vi "DeadbandFilter.vi"(8 "guardband value":dbl=0.1 format="%#_13g", 10 "JoystickAxis":dbl) -> (2 "FilteredJoystickAxis":dbl)   [LabVIEW 2017]
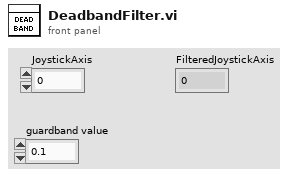
[diagram p1: front panel]
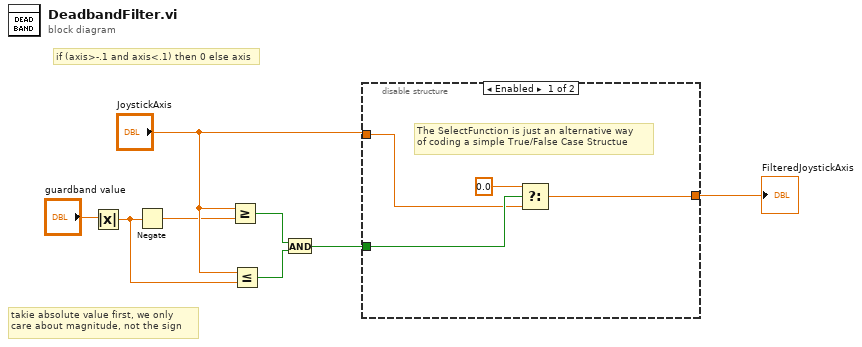
[diagram p0: block diagram]
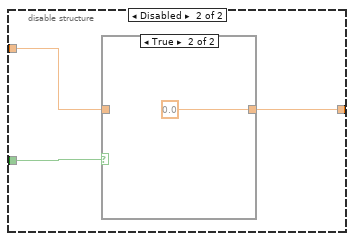
[diagram p2: hidden frame]
diagram:
  # "takie absolute value first, we only \ncare about magnitude, not the sign"
  # "if (axis>-.1 and axis<.1) then 0 else axis"
  n1 = Absolute Value(x="guardband value") -> (abs(x)=w1:dbl)
  n2 = Negate(x=w1) -> (-x=w2:dbl)
  n3 = Greater Or Equal?(x="JoystickAxis", y=w2) -> (x >= y?=w7:bool)
  n4 = Less Or Equal?(x="JoystickAxis", y=w1) -> (x <= y?=w8:bool)
  n5 = And(x=w7, y=w8) -> (x .and. y?=w6:bool)
  n6 = disable-structure shown="Enabled" {
    disable-tunnel: w6 -> [w10 w15]
    disable-tunnel: "JoystickAxis" -> [w9 w14]
    disable-tunnel: [w11 w13] -> w4
    frame Enabled {
      # "The SelectFunction is just an alternative way \nof coding a simple True/False Case Structue"
      n7 = Select(t=0.0, s=w10, f=w9) -> (s? t:f=w11:dbl)
    }
    frame Disabled {
      n8 = case shown="True" w15 {
        tunnel: [w16 0.0] -> w13
        tunnel: w14 -> [w16 _]
        frame False {
        }
        frame True {
        }
      }
    }
  }
  "FilteredJoystickAxis" <- w4
